vi "WordTable.vi"(8 "Error In":errorcluster, 11 "File Path Control":path) -> (0 "Error Out":errorcluster, 2 "待写入项2":string[](array[string]), 3 "待写入项":string[](array[string]))   [LabVIEW 2019]
uses:
  <vilib>/regexp/Match Regular Expression.xnode
panel:
  out "Text":string
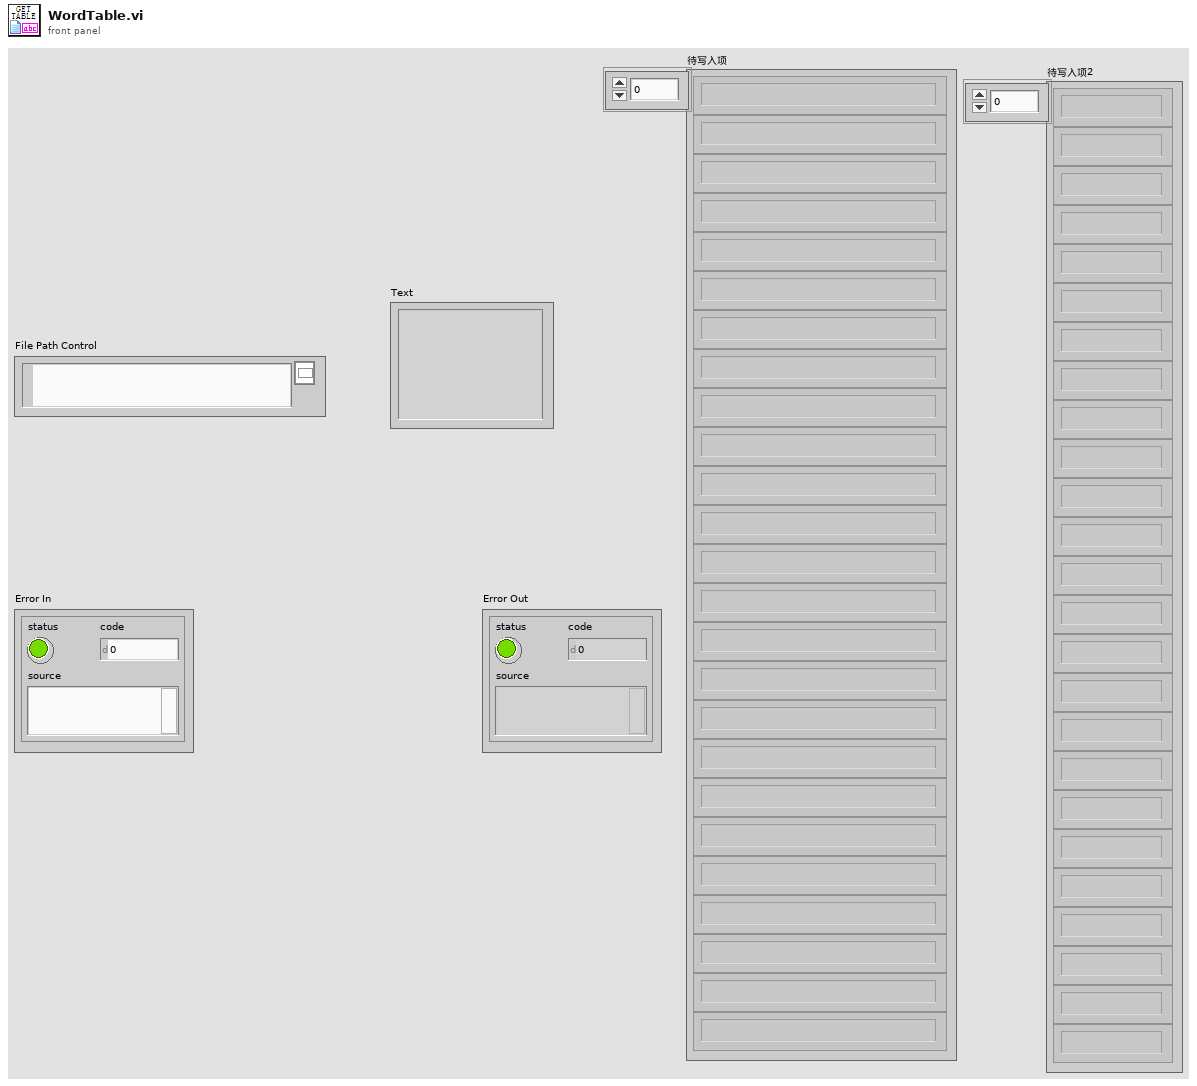
[diagram p1: front panel]
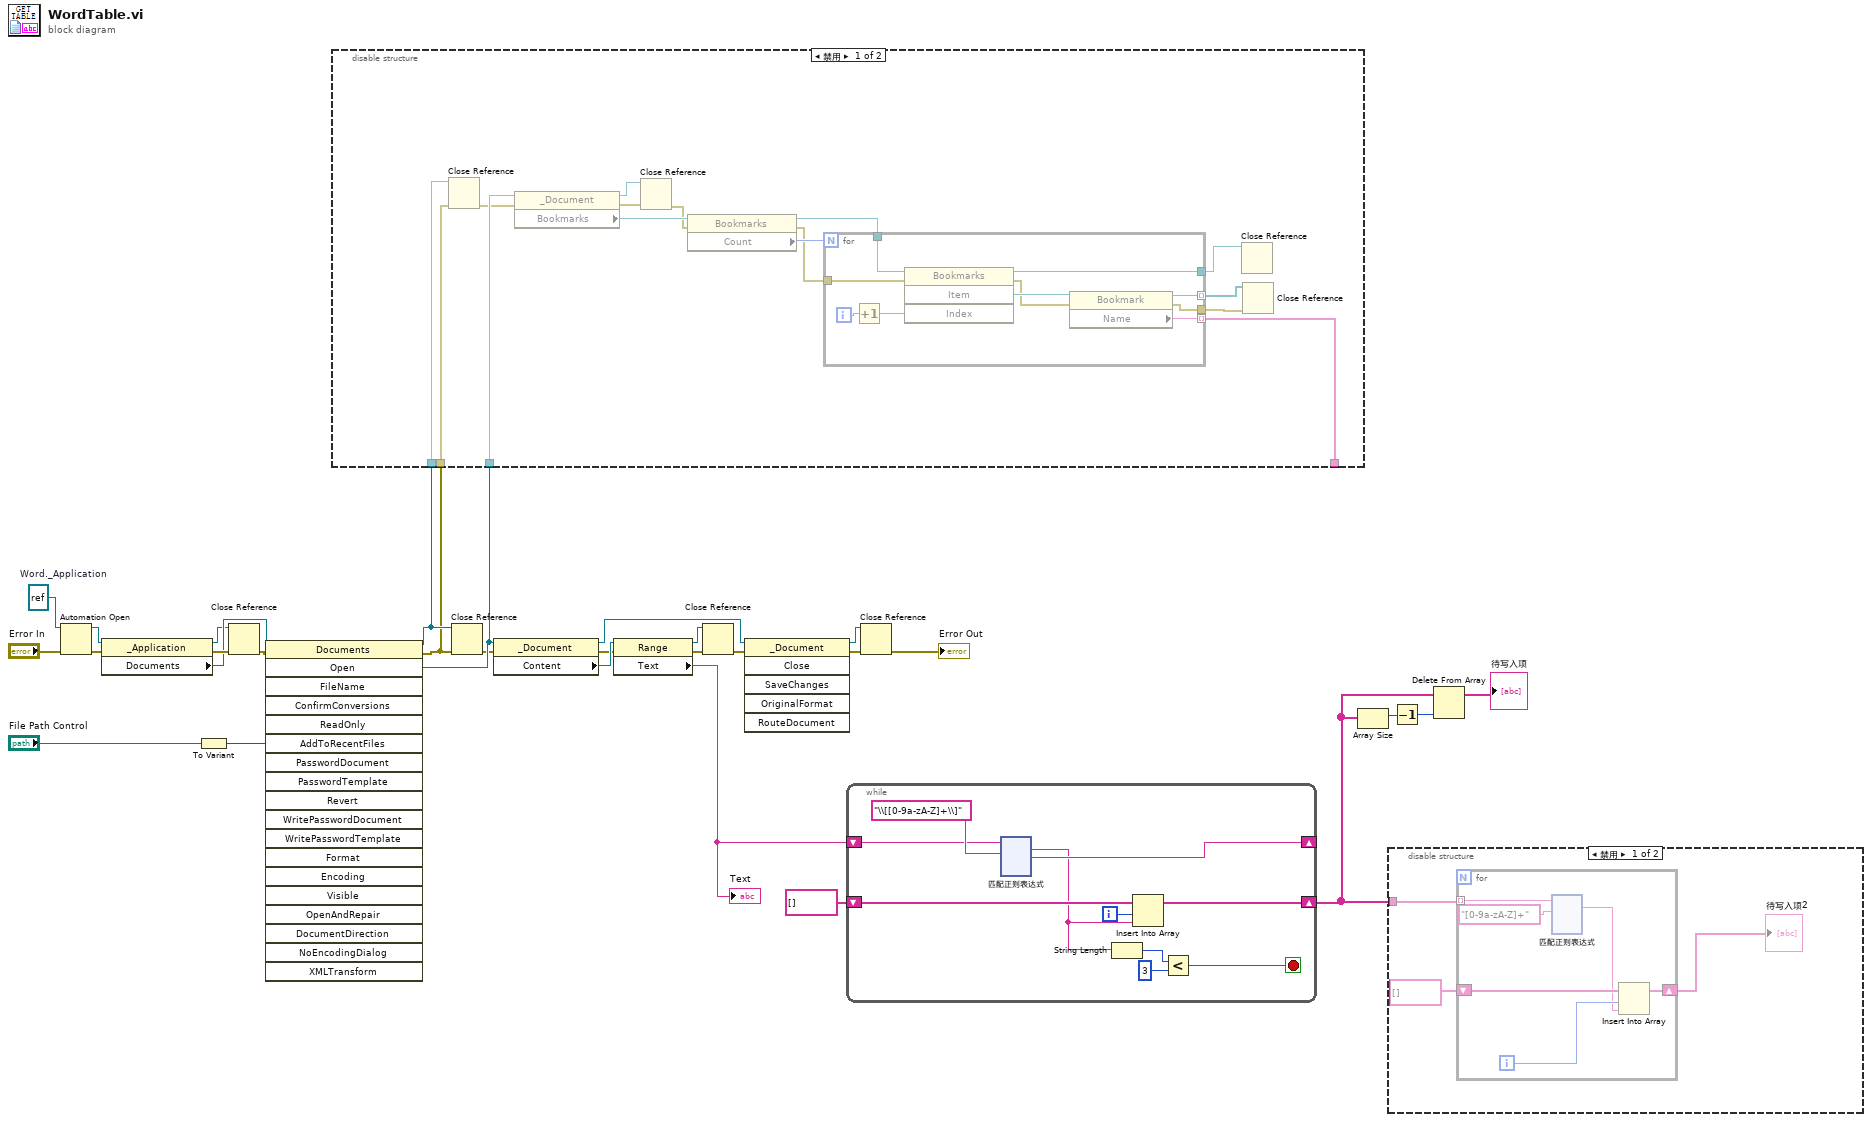
[diagram p0: block diagram]
diagram:
  w29 = refnum<k7> refnum  # Word._Application
  n1 = Automation Open(error in (no error)="Error In", Automation Refnum=w29) -> (Automation Refnum=w28:refnum<k7>, error out=w27:errorcluster)  [unwired: 2 in]
  n2 = property class="_Application"(reference=w28, error in=w27) -> (reference out=w21:refnum<k7>, error out=w26:errorcluster, "Documents"=w25:refnum<k7>)
  n3 = To Variant(anything="File Path Control") -> (Variant=w23:variant)
  n4 = Close Reference(reference=w21, error in (no error)=w26) -> (error out=w22:errorcluster)
  n5 = invoke class="Documents" method="Open"(reference=w25, error in=w22, "FileName"=w23) -> (reference out=w8:refnum<k7>, error out=w7:errorcluster, "Open"=w19:refnum<k7>)  [unwired: 16 in, 16 out]
  n6 = disable-structure shown="禁用" {
    disable-tunnel: w19 -> [w44 _]
    disable-tunnel: [w43 _] -> _
    disable-tunnel: w8 -> [w42 _]
    disable-tunnel: w7 -> [w41 _]
    frame Disabled {
      n7 = Close Reference(reference=w42, error in (no error)=w41) -> (error out=w30:errorcluster)
      n8 = property on="属性节点" class="_Document"(reference=w44, error in=w30) -> (reference out=w37:refnum<k7>, error out=w36:errorcluster, "Bookmarks"=w38:refnum<k7>)
      n9 = Close Reference(reference=w37, error in (no error)=w36) -> (error out=w35:errorcluster)
      n10 = property on="属性节点" class="Bookmarks"(reference=w38, error in=w35) -> (reference out=w39:refnum<k7>, error out=w34:errorcluster, "Count"=w40:i32)
      n11 = for {
        N: w40 -> [_]
        tunnel: w39 -> [w54]
        tunnel: [w50] -> w43 mode=indexing
        tunnel: w34 -> [w49]
        tunnel: [w48] -> w33 mode=indexing
        tunnel: [w47] -> w32
        tunnel: [w45] -> w31
        i -> [w53]
        n12 = Increment(x=w53) -> (x+1=w52:i32)
        n13 = invoke on="调用节点" class="Bookmarks" method="Item"(reference=w54, error in=w49, "Index"=w52) -> (reference out=w45:refnum<k7>, error out=w46:errorcluster, "Item"=w51:refnum<k7>)  [unwired: 1 in, 1 out]
        n14 = property on="属性节点" class="Bookmark"(reference=w51, error in=w46) -> (reference out=w48:refnum<k7>, error out=w47:errorcluster, "Name"=w50:string)
      }
      n15 = Close Reference(reference=w31) -> ()  [unwired: 1 in, 1 out]
      n16 = Close Reference(reference=w33, error in (no error)=w32) -> ()  [unwired: 1 out]
    }
    frame Enabled {
    }
  }
  n17 = Close Reference(reference=w8, error in (no error)=w7) -> (error out=w10:errorcluster)
  n18 = property class="_Document"(reference=w19, error in=w10) -> (reference out=w13:refnum<k7>, error out=w17:errorcluster, "Content"=w18:refnum<k7>)
  n19 = property class="Range"(reference=w18, error in=w17) -> (reference out=w15:refnum<k7>, error out=w16:errorcluster, "Text"=w6:string)
  "Text" <- w6
  n20 = Close Reference(reference=w15, error in (no error)=w16) -> (error out=w14:errorcluster)
  n21 = invoke class="_Document" method="Close"(reference=w13, error in=w14) -> (reference out=w11:refnum<k7>, error out=w12:errorcluster)  [unwired: 4 in, 4 out]
  n22 = while {
    shift-right: [w60] -> _
    shift-left: w6 -> [w59]
    shift-right: [w62] -> w3
    shift-left: string[] [] -> [w63]
    i -> [w61]
    stop <- w56 stop-if-true
    n23 = xnode "匹配正则表达式"("输入字符串"=w59, "正则表达式"="\\[[0-9a-zA-Z]+\\]") -> ("所有匹配"=w55:string, "匹配之后"=w60:string)  [unwired: 4 in, 3 out]
    n24 = String Length(string=w55) -> (length=w58:i32)
    n25 = Insert Into Array(array=w63, index=w61, new element=w55) -> (w62:string[])
    n26 = Less?(x=w58, y=3) -> (x < y?=w56:bool)
  }
  n27 = Close Reference(reference=w11, error in (no error)=w12) -> (error out=→"Error Out":errorcluster)
  n28 = Array Size(array=w3) -> (size(s)=w2:i32)
  n29 = disable-structure shown="禁用" {
    disable-tunnel: w3 -> [w179 _]
    frame Disabled {
      n30 = for {
        tunnel: w179 -> [w187] mode=indexing
        shift-right: [w183] -> w180
        shift-left: string[] [] -> [w184]
        i -> [w185]
        n31 = xnode "匹配正则表达式"("输入字符串"=w187, "正则表达式"="[0-9a-zA-Z]+") -> ("所有匹配"=w182:string)  [unwired: 4 in, 4 out]
        n32 = Insert Into Array(array=w184, index=w185, new element=w182) -> (w183:string[])
      }
      "待写入项2" <- w180
    }
    frame Enabled {
    }
  }
  n33 = Decrement(x=w2) -> (x-1=w1:i32)
  n34 = Delete From Array(array=w3, index=w1) -> (array with subset deleted=→"待写入项":string[])  [unwired: 1 in, 1 out]
